vi "PH_Stepmotor_BaseClass.set i Attributes and open DIM Servives.vi"(2 "error in":errorcluster, 3 "Instance Name":string) -> (0 "error out":errorcluster, 1 "i Attribute":T1 {"Axes PSDB Thread"."Data Status" items=["no info", "no Data collection", "no problem", "Error getting the ID", "Error writing Data", "Error getting the subsystem", "Error getting the Shot ID", "Error getting the Shot Types", "Error getting the Experiments", "Error verifying wanted Shottype", "Error verifying wanted Experiment"]})   [LabVIEW 2014, in "PH_Stepmotor_BaseClass.lvlib"]
uses:
  PH_Stepmotor_BaseClass.lvlib
  PH_Stepmotor_BaseClass.i attribute.ctl
  PH_PSDBWriter/PH_PSDBWriter.Data Status.ctl
  PH_Stepmotor_BaseClass.Axis Attributes.ctl
  PH_Stepmotor_BaseClass.Axis Settings.ctl
  PH_Stepmotor_BaseClass.Motor Type.ctl
  PH_Stepmotor_BaseClass.Axis DIM Service IDs.ctl
  PH_Stepmotor_BaseClass.Axis Activity.ctl
  PH_Stepmotor_BaseClass.GUI Refs.ctl
  PH_AxisGUI_BaseClass/PH_AxisGUI_BaseClass.lvlib
  PH_PSDBWriter/PH_PSDBWriter.lvlib
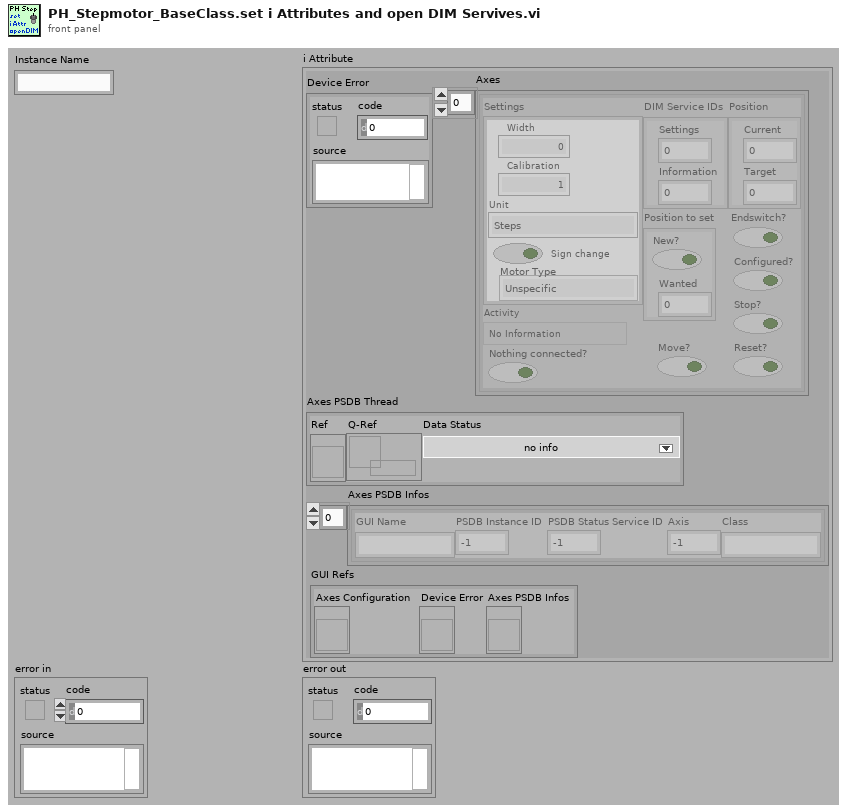
[diagram p1: front panel]
types:
  T1 = typedef "PH_Stepmotor_BaseClass.lvlib/PH_Stepmotor_BaseClass.i attribute.ctl" = cluster{"Device Error":errorcluster, "Axes PSDB Thread":cluster{"Ref":refnum<vi>, "Q-Ref":refnum<queue>, "Data Status":T2}, "Axes":T3[], "Axes PSDB Infos":cluster{"GUI Name":string, "PSDB Instance ID":i32, "PSDB Status Service ID":i32, "Axis":i32, "Class":string}[], "GUI Refs":T8}
  T2 = typedef "PH_PSDBWriter.lvlib/PH_PSDBWriter.Data Status.ctl" = i16
  T3 = typedef "PH_Stepmotor_BaseClass.lvlib/PH_Stepmotor_BaseClass.Axis Attributes.ctl" = cluster{"Settings":T4, "Endswitch?":bool, "DIM Service IDs":T6, "Activity":T7, "Configured?":bool, "Position":cluster{"Current":i32, "Target":i32}, "Position to set":cluster{"New?":bool, "Wanted":i32}, "Stop?":bool, "Reset?":bool, "Move?":bool, "Nothing connected?":bool}
  T4 = typedef "PH_Stepmotor_BaseClass.lvlib/PH_Stepmotor_BaseClass.Axis Settings.ctl" = cluster{"Sign change":bool, "Width":dbl, "Calibration":dbl, "Unit":string, "Motor Type":T5, "Unit Width":string, "Unit CF":string}
  T5 = typedef "PH_Stepmotor_BaseClass.lvlib/PH_Stepmotor_BaseClass.Motor Type.ctl" = enum16{"Unspecific", "OWIS 49.120.2633", "OWIS 49.060.1033", "OWIS 43.040.2558", "Diamond Motion 2200 series", "OWIS 49.120.266B.MV6", "Calorimeter", "Linear Stage 1", "MICOS VT-80", "MICOS VT-80 S", "Standa Rotstage nt0.95A", "PUF RA 320.200", "PUF RA 800.200", "PUF RA 800.400", "PUF RA 400.50", "1324.nn.800.50", "1324.n9c.800.50", "1324.nn.320.200", "1324.nn.400.200", "1324.nn.800.200", "1324.nn.400.50", "1324.8c9c.800.50", "1324.8c9c.400.200"}
  T6 = typedef "PH_Stepmotor_BaseClass.lvlib/PH_Stepmotor_BaseClass.Axis DIM Service IDs.ctl" = cluster{"Settings":i32, "Information":i32}
  T7 = typedef "PH_Stepmotor_BaseClass.lvlib/PH_Stepmotor_BaseClass.Axis Activity.ctl" = enum16{"No Information", "stopped", "running", "Failure", "Alarm", "stopped at backward ES", "stopped at foreward ES"}
  T8 = typedef "PH_Stepmotor_BaseClass.lvlib/PH_Stepmotor_BaseClass.GUI Refs.ctl" = cluster{"Axes Configuration":refnum<vi>, "Device Error":refnum<vi>, "Axes PSDB Infos":refnum<vi>}
  T9 = cluster{"Name":string, "PSDB Instance ID":i32, "PSDB Status Service ID":i32, "Axis":i32, "Class":string}
  T10 = typedef "PH_Stepmotor_BaseClass.lvlib/PH_Stepmotor_BaseClass.Axis Address.ctl" = cluster{"Instance":string, "Motor Nr":i32}
  T11 = cluster{"Address":T10, "GUI Class":string, "GUI Instance":string}[]
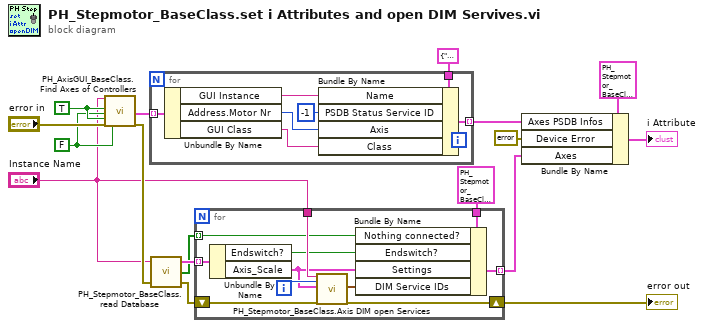
[diagram p0: block diagram]
diagram:
  w8 = FALSE ("PH_Sixpack_Switch")
  w10 = TRUE ("PH_AxisGUI_6P")
  n1 = call "PH_AxisGUI_BaseClass.Find Axes of Controllers.vi"("Own Motion Instance (N/A)"="Instance Name", "PH_AxisGUI_6P"=w10, "PH_Sixpack_Switch"=w8, "PH_Waveplate-GUI_6P"=w10, "error in"="error in", "PH_4_Pos_Selector"=w8) -> ("Result"=w2:T11, "error out"=w7:errorcluster)  [unwired: 12 in]
  n2 = for {
    tunnel: T9 {"Name"="", "PSDB Instance ID"=0, "PSDB Status Service ID"=-1, "Axis"=0, "Class"=""} ("Axis PSDB Information") -> [w24]
    tunnel: [w23] -> w13 mode=indexing
    tunnel: w2 -> [w21] mode=indexing
    n3 = Unbundle By Name(w21) -> ("GUI Instance"=w20:string, "Address.Motor Nr"=w19:i32, "GUI Class"=w18:string)
    n4 = Bundle By Name(cluster=w24, "Name"=w20, "PSDB Status Service ID"=-1 ("BSDB Status Service ID"), "Axis"=w19, "Class"=w18) -> (w23:T9)
  }
  n5 = call "PH_Stepmotor_BaseClass.read Database.vi"("error in (no error)"=w7, "DB Entry to read"="Instance Name") -> ("error out"=w5:errorcluster, "Entry empty?"=w1:bool[], "Axes Data"=w3:cluster{"Axis_Scale":T4, "Endswitch?":bool}[])  [unwired: 1 in]
  n6 = for {
    shift-right: [w33] -> w6
    shift-left: w5 -> [w29]
    tunnel: "Instance Name" -> [w31]
    tunnel: T3 {"Settings"={"Sign change"=FALSE, "Width"=0.0, "Calibration"=0.0, "Unit"="", "Motor Type"=enum."Unspecific", "Unit Width"="", "Unit CF"=""}, "Endswitch?"=FALSE, "DIM Service IDs"={"Settings"=0, "Information"=0}, "Activity"=enum."No Information", "Configured?"=FALSE, "Position"={"Current"=0, "Target"=0}, "Position to set"={"New?"=FALSE, "Wanted"=0}, "Stop?"=FALSE, "Reset?"=FALSE, "Move?"=FALSE, "Nothing connected?"=FALSE} ("motor") -> [w34]
    tunnel: [w35] -> w11 mode=indexing
    tunnel: w3 -> [w30] mode=indexing
    tunnel: w1 -> [w25] mode=indexing
    i -> [w32]
    n7 = Unbundle By Name(w30) -> ("Endswitch?"=w26:bool, "Axis_Scale"=w27:T4)
    n8 = call "PH_Stepmotor_BaseClass.Axis DIM open Services.vi"("Instancename"=w31, "Axis Number"=w32, "Axis Settings"=w27, "error in (no error)"=w29) -> ("Axis DIM Service IDs"=w28:T6, "error out"=w33:errorcluster)  [unwired: 14 in]
    n9 = Bundle By Name(cluster=w34, "Nothing connected?"=w25, "Endswitch?"=w26, "Settings"=w27, "DIM Service IDs"=w28) -> (w35:T3)
  }
  "error out" <- w6
  n10 = Bundle By Name(cluster=T1 {"Device Error"={"status"=FALSE, "code"=0, "source"=""}, "Axes PSDB Thread"={"Ref"=refnum, "Q-Ref"=refnum, "Data Status"=0}, "Axes"=[], "Axes PSDB Infos"=[], "GUI Refs"={"Axes Configuration"=refnum, "Device Error"=refnum, "Axes PSDB Infos"=refnum}} ("i Attribute"), "Axes PSDB Infos"=w13, "Device Error"=errorcluster {"status"=FALSE, "code"=0, "source"=""}, "Axes"=w11) -> (→"i Attribute":T1)
